vi "Autotest.vi"(8 "error in (no error)":errorcluster caption="entrée d'erreur (pas d'erreur)", 11 "Class Camera IV3-500CA en entrée":refnum<class "Class Camera IV3-500CA.lvclass">) -> (0 "error out":errorcluster caption="sortie d'erreur", 2 "Autotest":bool, 3 "Class Camera IV3-500CA en sortie":refnum<class "Class Camera IV3-500CA.lvclass">)   [LabVIEW 2020, in "Library Instrument & Equipement.lvlib" / "Library Camera.lvlib" / "Class Camera IV3-500CA.lvclass"]
uses:
  Class Camera IV3-500CA.lvclass
  Class Camera  IV3-500CA - Read version/Class Camera  IV3-500CA - Read version.lvclass
  Class Camera IV3-500CA.lvclass/Class Camera IV3-500CA.ctl
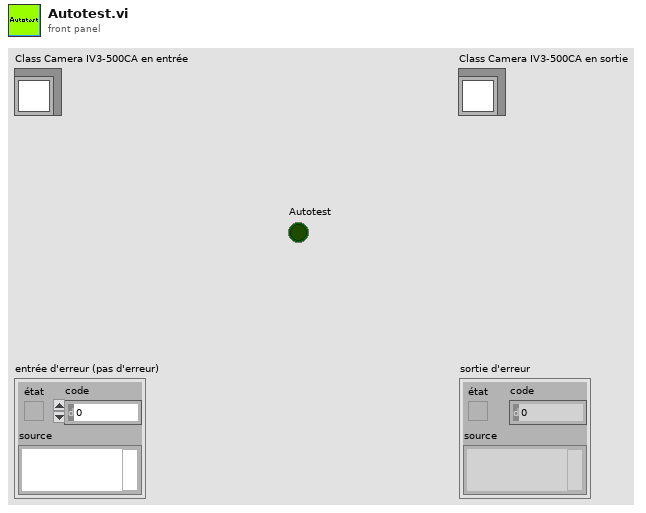
[diagram p1: front panel]
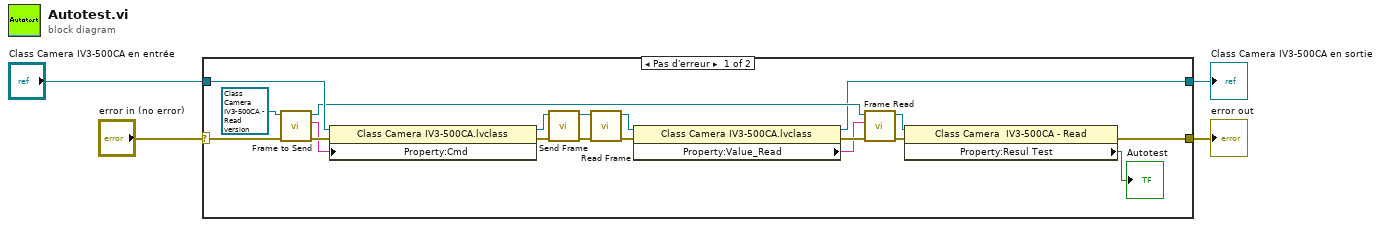
[diagram p0: block diagram]
diagram:
  n1 = case shown="Pas d'erreur" "error in (no error)" {
    selector: "error in (no error)" -> [w14 w25]
    tunnel: [w22 w25] -> w3
    tunnel: [w6 w24] -> w1
    tunnel: "Class Camera IV3-500CA en entrée" -> [w13 w24]
    frame No Error {
      n2 = call-dynamic "Frame to Send.vi"("error in (no error)"=w14, "Class Camera  IV3-500CA - Start Program en Entrée"=refnum<class "Class Camera  IV3-500CA - Read version.lvclass"> refnum ("Library Camera.lvlib:Class Camera  IV3-500CA - Read version.lvclass")) -> ("error out"=w20:errorcluster, "Frame to Write"=w19:string, "Class Camera  IV3-500CA - Start Program en Sortie"=w10:refnum<class "Class Camera  IV3-500CA - Read version.lvclass">)  [unwired: 7 in]
      n3 = property class="Class Camera IV3-500CA.lvclass"(reference=w13, error in=w20, "Property:Cmd"=w19) -> (reference out=w18:refnum<class "Class Camera IV3-500CA.lvclass">, error out=w21:errorcluster)
      n4 = call-dynamic "Send Frame.vi"("error in (no error)"=w21, "Class Camera IV3-500CA (Default) en Entrée"=w18) -> ("error out"=w17:errorcluster, "Class Camera IV3-500CA (Default) en Sortie"=w16:refnum<class "Class Camera IV3-500CA.lvclass">)  [unwired: 8 in]
      n5 = call-dynamic "Read Frame.vi"("error in (no error)"=w17, "Class Camera IV3-500CA (Default) en Entrée"=w16) -> ("error out"=w12:errorcluster, "Class Camera IV3-500CA (Default) en Sortie"=w8:refnum<class "Class Camera IV3-500CA.lvclass">)  [unwired: 8 in]
      n6 = property class="Class Camera IV3-500CA.lvclass"(reference=w8, error in=w12) -> (reference out=w6:refnum<class "Class Camera IV3-500CA.lvclass">, error out=w9:errorcluster, "Property:Value_Read"=w7:string)
      n7 = call-dynamic "Frame Read.vi"("error in (no error)"=w9, "Frame Read"=w7, "Class Camera  IV3-500CA - Start Program en Entrée"=w10) -> ("error out"=w11:errorcluster, "Class Camera  IV3-500CA - Start Program en Sortie"=w5:refnum<class "Class Camera  IV3-500CA - Read version.lvclass">)  [unwired: 7 in]
      n8 = property class="Class Camera  IV3-500CA - Read "(reference=w5, error in=w11) -> (error out=w22:errorcluster, "Property:Resul Test "=→"Autotest":bool)  [unwired: 1 out]
    }
    frame Error {
    }
  }
  "error out" <- w3
  "Class Camera IV3-500CA en sortie" <- w1
